vi "find_template_test.vi"() -> ()   [LabVIEW 2024]
uses:
  find_template parameters.ctl
  find_template_output_parameters.ctl
  Vision.lvlib
panel:
  out "Templates":T1
  in  "find_template parameters":T2
  out "log out":string
  in  "Field of View":cluster{"fieldOfViewX":sgl, "fieldOfViewY":sgl}={"fieldOfViewX"=1.4, "fieldOfViewY"=1.048}
  in  "Target Path":path=path "C:/Users/cfang/Desktop/pixel-gantry-control/Data/HDI_fid.png"
  out "error out":errorcluster
  out "Image":T3(plugin-control)
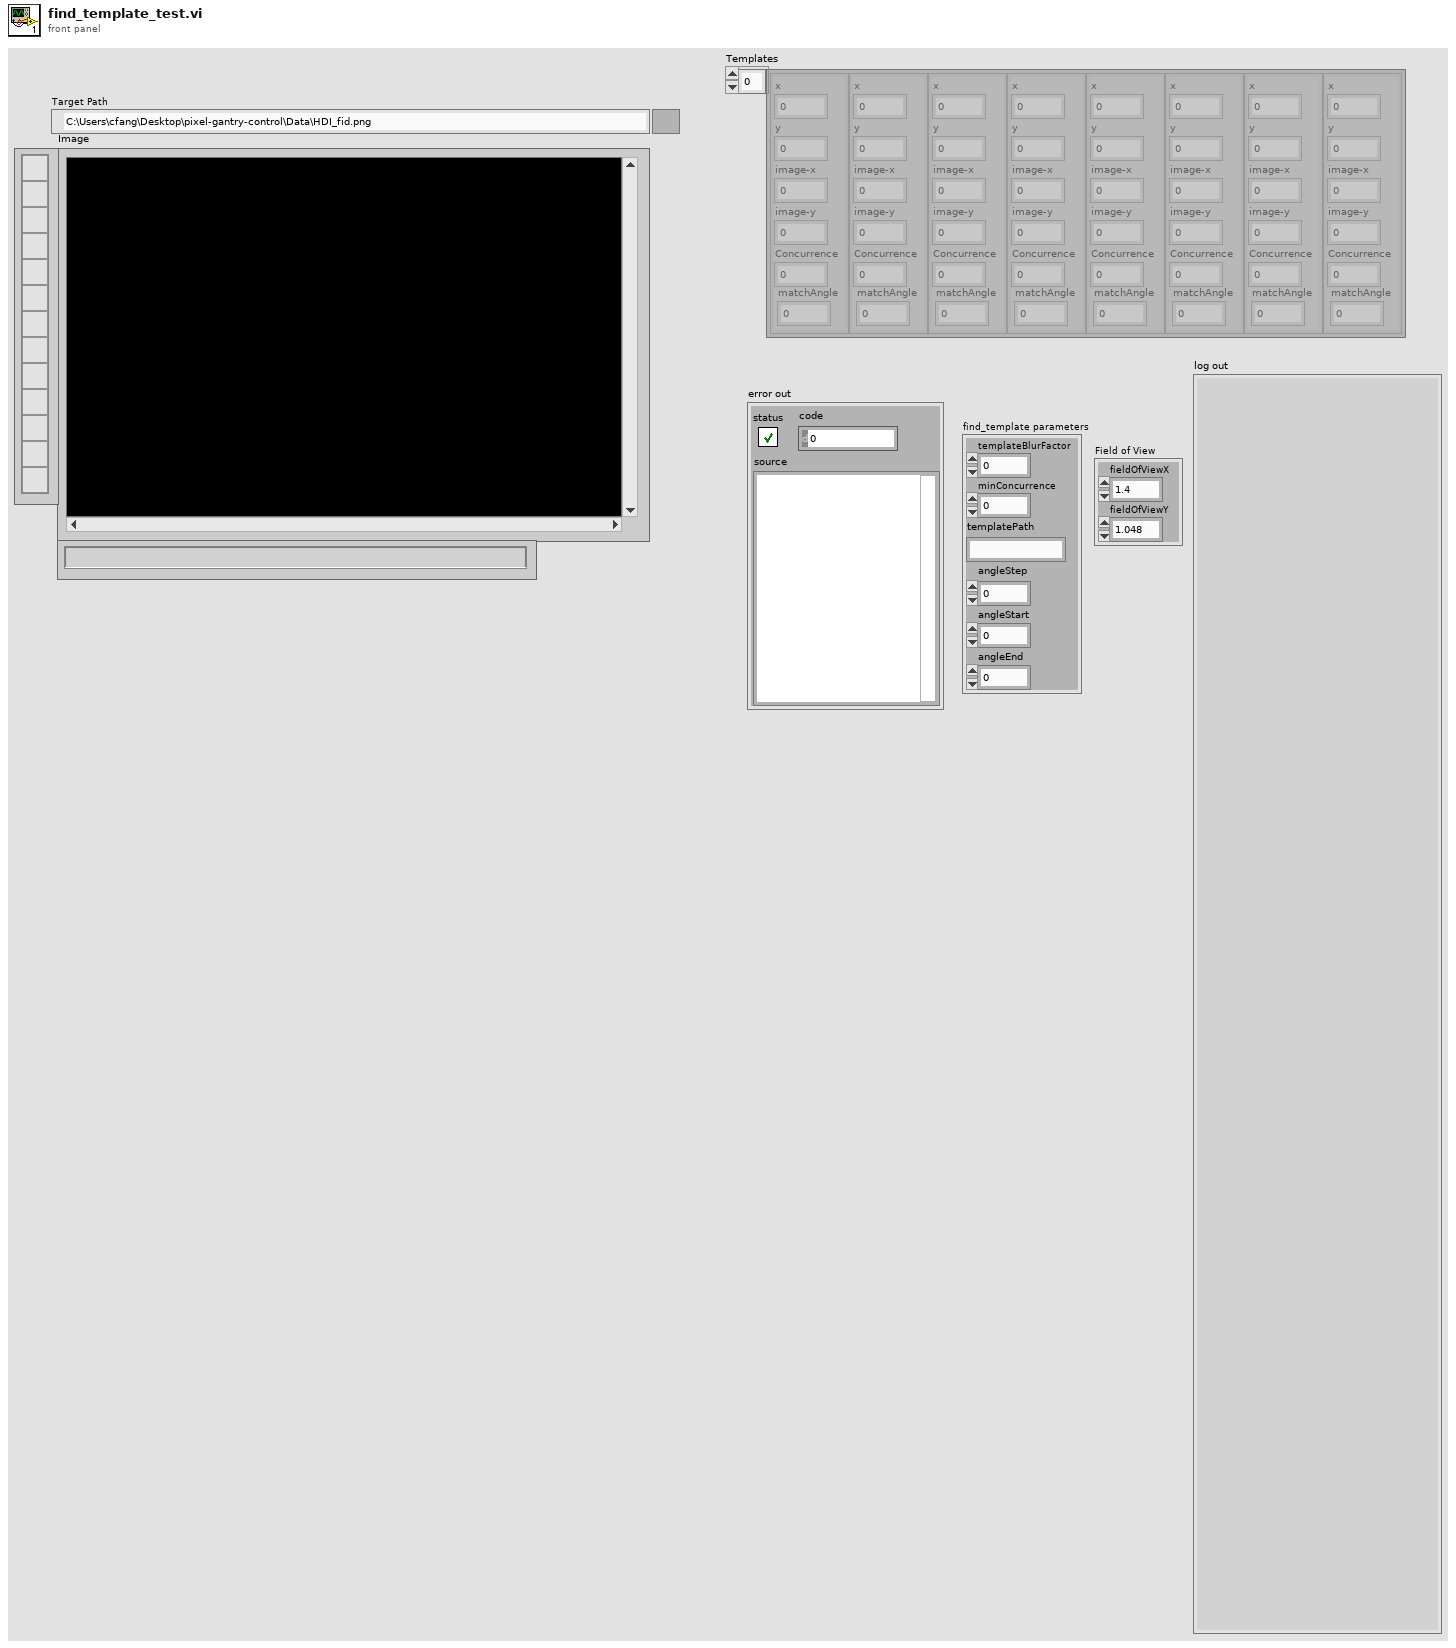
[diagram p1: front panel]
types:
  T1 = typedef "find_template_output_parameters.ctl" = cluster{"x":dbl, "y":dbl, "image-x":dbl, "image-y":dbl, "Concurrence":dbl, "matchAngle":dbl}[]
  T2 = typedef "Vision.lvlib/find_template parameters.ctl" = cluster{"templateBlurFactor":i32, "minConcurrence":sgl, "templatePath":string, "angleStep":dbl, "angleStart":dbl, "angleEnd":dbl}
  T3 = typedef "IMAQ Image.ctl" = refnum<image>
  T4 = cluster{"Left":i32, "Top":i32, "Right":i32, "Bottom":i32}
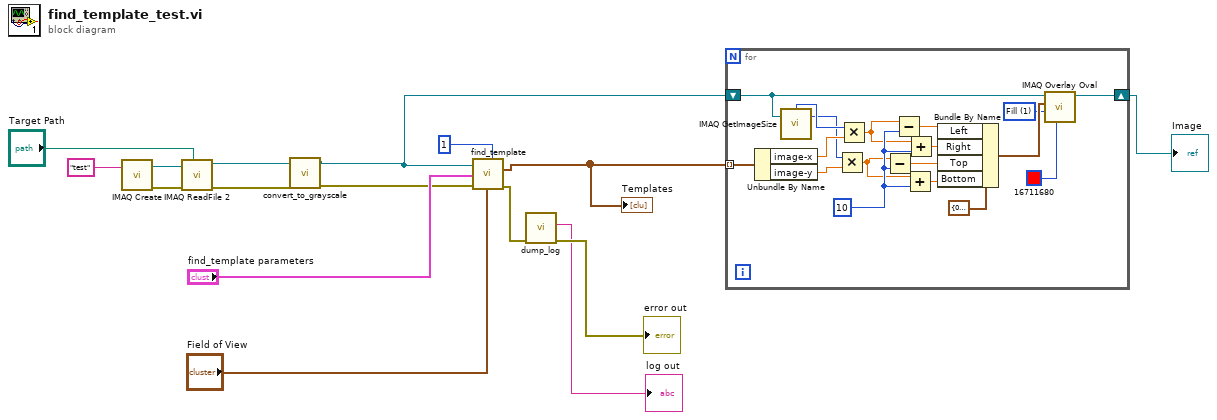
[diagram p0: block diagram]
diagram:
  n1 = call "IMAQ Create"("Image Name"="test") -> ("New Image"=w16:T3, "error out"=w14:errorcluster)  [unwired: 4 in]
  n2 = call "IMAQ ReadFile 2"("File Path"="Target Path", "error in (no error)"=w14, "Image"=w16) -> ("error out"=w4:errorcluster, "Image Out"=w2:T3)  [unwired: 4 in, 3 out]
  n3 = call "convert_to_grayscale.vi"("error in (no error)"=w4, "Image in"=w2) -> ("error out"=w3:errorcluster, "Image out"=w1:T3)  [unwired: 8 in]
  n4 = call "find_template.vi"("Shrink Factor"=1, "Field of View"="Field of View", "error in"=w3, "find_template parameters"="find_template parameters", "Image"=w1) -> ("error out"=w9:errorcluster, "Matches"=w5:T1)  [unwired: 5 in]
  "Templates" <- w5
  n5 = call "dump_log.vi"("error in (no error)"=w9) -> ("error out"=→"error out":errorcluster, "log out"=→"log out":string)  [unwired: 9 in]
  n6 = for {
    tunnel: w5 -> [w34] mode=indexing
    shift-right: [w18] -> w12
    shift-left: w1 -> [w29]
    w17 = u32 1 items=["Frame", "Fill"] ("Drawing Mode (Frame)")
    w22 = 10
    n7 = Unbundle By Name(w34) -> ("image-x"=w33:dbl, "image-y"=w31:dbl)
    n8 = call "IMAQ GetImageSize"("Image"=w29) -> ("Y Resolution"=w30:i32, "X Resolution"=w32:i32)  [unwired: 3 in, 1 out]
    n9 = Multiply(x=w30, y=w31) -> (x*y=w21:dbl)
    n10 = Multiply(x=w32, y=w33) -> (x*y=w20:dbl)
    n11 = Subtract(x=w21, y=w22) -> (x-y=w23:dbl)
    n12 = Subtract(x=w20, y=w22) -> (x-y=w24:dbl)
    n13 = Add(x=w21, y=w22) -> (x+y=w25:dbl)
    n14 = Add(x=w20, y=w22) -> (x+y=w26:dbl)
    n15 = Bundle By Name(cluster=T4 {"Left"=0, "Top"=0, "Right"=0, "Bottom"=0} ("Bounding Rectangle"), "Left"=w24, "Right"=w26, "Top"=w23, "Bottom"=w25) -> (w19:T4)
    n16 = call "IMAQ Overlay Oval"("Color"=u32 16711680, "Drawing Mode (Frame)"=w17, "Bounding Rectangle"=w19, "Image"=w29) -> ("Image Out"=w18:T3)  [unwired: 6 in, 1 out]
  }
  "Image" <- w12
